vi "Get FIFO Data.vi"(6 "offset":i32, 8 "error in (no error)":errorcluster, 11 "bitfile xml in":string) -> (0 "error out":errorcluster, 2 "HostToTargetFIFOs":T1[](array[typedef]), 3 "TargetToHost FIFOs":T1[](array[typedef]), 4 "offset past EndTag":i32)   [LabVIEW 2010, in "FPGA Bitfile Utility.lvlib"]
uses:
  <userlib>/_FPGA Interface Advanced Tools/FPGA Bitfile Utility/FPGA Bitfile Utility.lvlib
  <userlib>/_FPGA Interface Advanced Tools/FPGA Bitfile Utility/TypeDefs/FIFO Info.ctl
  <vilib>/rvi/DataTransferAndStorage/Container/Common/niFpgaDataTypeControl.ctl
  <vilib>/rvi/Utilities/XML/nirviXML_GetValue.vi
  <vilib>/rvi/Utilities/XML/nirviXML_GetValue_String.vi
  resource/RVI/compilationResultUtilities/niLvFpgaGetDmaChannelInfoFromXML.vi
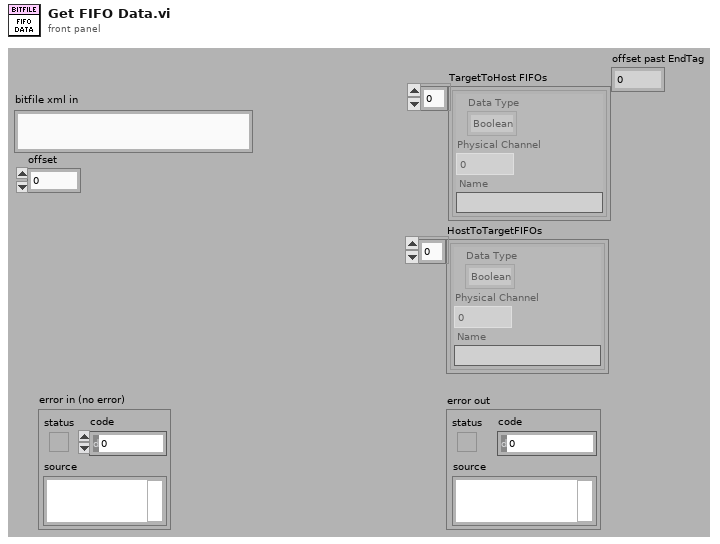
[diagram p1: front panel]
types:
  T1 = typedef "FPGA Bitfile Utility.lvlib/FIFO Info.ctl" = cluster{"Data Type":T2, "Physical Channel":u32, "Name":string}
  T2 = typedef "niFpgaDataTypeControl.ctl" = enum32{"Boolean", "I8", "I16", "I32", "I64", "U8", "U16", "U32", "U64", "FXP", "CustomControl"}
  T3 = cluster{"Data Type":T2, "Physical Channel":u32, "Name":string}[]
  T4 = typedef "Fifo_DMA_Config.ctl" = cluster{"Name":string, "Depth":u32, "Write? (Deprecated:Use Implementation)":bool, "Physical Channel":u32, "Base Address":u32, "Data Width":u32, "Data Type":T2, "FXP Properties":variant, "Write Window Address":u32, "Implementation":T5, "Control Set":u32}
  T5 = typedef "niFpgaDmaChannelImplementation.ctl" = enum16{"niFpgaTargetToHost", "niFpgaHostToTarget", "niFpgaPeerToPeerWriter", "niFpgaPeerToPeerReader", "niCoreTargetToHost", "niCoreHostToTarget"}
  T6 = cluster{"Data Type":T2, "Physical Channel":u32, "Name":string}
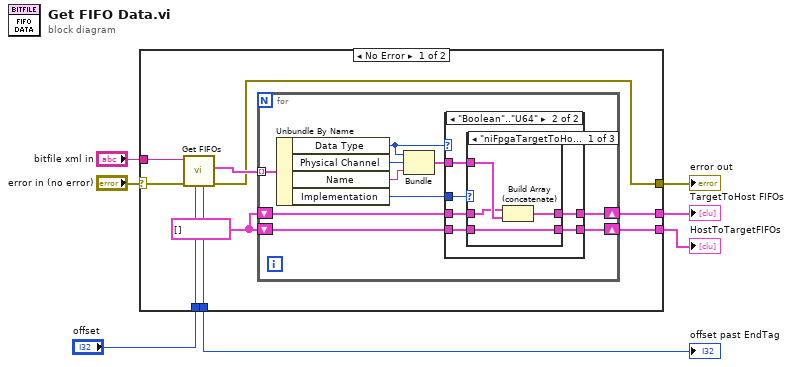
[diagram p0: block diagram]
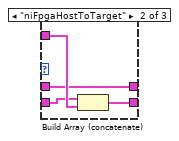
[diagram p3: hidden frame]
diagram:
  n1 = case shown="No Error" "error in (no error)" {
    selector: "error in (no error)" -> [w12 w46]
    tunnel: [w11 w46] -> w6
    tunnel: [w15 _] -> w5
    tunnel: [w14 _] -> w4
    tunnel: "bitfile xml in" -> [w10 _]
    tunnel: "offset" -> [w9 w45]
    tunnel: [w8 w45] -> w1
    frame No Error {
      w16 = T3 []
      n2 = call <userlib>:"Get FIFOs.vi"("offset"=w9, "error in (no error)"=w12, "bitfile xml in"=w10) -> ("error out"=w11:errorcluster, "DMA configuration array"=w13:T4[], "offset past EndTag"=w8:i32)  [unwired: 6 in]
      n3 = for {
        tunnel: w13 -> [w26] mode=indexing
        shift-right: [w20] -> w15
        shift-left: w16 -> [w19]
        shift-right: [w18] -> w14
        shift-left: w16 -> [w17]
        n4 = Unbundle By Name(w26) -> ("Data Type"=w25:T2, "Physical Channel"=w24:u32, "Name"=w23:string, "Implementation"=w21:T5)
        n5 = Bundle("Data Type"=w25, "Physical Channel"=w24, "Name"=w23) -> (w22:T6)  [unwired: 1 in]
        n6 = case shown="\"Boolean\"..\"U64\"" w25 {
          tunnel: w22 -> [_ w33]
          tunnel: w21 -> [_ w34]
          tunnel: [w28 w32] -> w20
          tunnel: w19 -> [w28 w31]
          tunnel: [w27 w30] -> w18
          tunnel: w17 -> [w27 w29]
          frame Default {
          }
          frame "Boolean".."U64" {
            n7 = case shown="\"niFpgaTargetToHost\"" w34 {
              tunnel: w33 -> [w38 w42 _]
              tunnel: [w37 w39 w44] -> w32
              tunnel: w31 -> [w36 w39 w44]
              tunnel: [w35 w41 w43] -> w30
              tunnel: w29 -> [w35 w40 w43]
              frame "niFpgaTargetToHost" {
                n8 = Build Array (concatenate)(w36, w38) -> (w37:T3)
              }
              frame "niFpgaHostToTarget" {
                n9 = Build Array (concatenate)(w40, w42) -> (w41:T3)
              }
              frame Default {
              }
            }
          }
        }
      }
    }
    frame Error {
    }
  }
  "error out" <- w6
  "TargetToHost FIFOs" <- w5
  "HostToTargetFIFOs" <- w4
  "offset past EndTag" <- w1
